vi "Update_Ch_Discription_client.vi"(1 "Channels to update In":T1[](array[typedef]) {"Duty" format="%016b"; "D" format="%#_5g"; "C" format="%#_5g"; "B" format="%#_5g"; "A" format="%#_5g"}) -> ()   [LabVIEW 2016]
doc: "This is an example of using features of the VI Server as a client. It shows how you might browse from one or more applications that may be exporting data from one or more data stations. \n\nThe example shows how to query a server for its list of exported VIs, how to get references to the VIs, and how call them with the Call By Reference function."
uses:
  Anemometry/Anemometry Sub Vis/Globals/Preference_global.vi
  Anemometry/Anemometry Sub Vis/Controls/Global_mode.ctl
  Sub VIs/ADAM Controls/Module_type_ADAM.ctl
  Sub VIs/ADAM Controls/Function_ADAM.ctl
  Sub VIs/ADAM Controls/Calib_type_ADAM.ctl
  Sub VIs/ADAM Controls/Address.ctl
  Sub VIs/ADAM Controls/Ch_description_ADAM.ctl
  Sub VIs/ADAM Controls/Channel_State.ctl
panel:
  in  "Server type":refnum<vi>
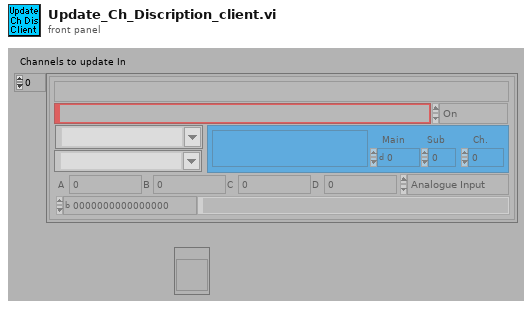
[diagram p1: front panel]
types:
  T1 = typedef "Ch_description_ADAM.ctl" = cluster{"Ch Name":string, "Type":T2, "Function":T3, "Ch State":T4, "Calibration type":T5, "A":dbl, "B":dbl, "C":dbl, "D":dbl, "Comments":string, "Address":T6, "String":string, "Duty":u16}
  T2 = typedef "Module_type_ADAM.ctl" = string
  T3 = typedef "Function_ADAM.ctl" = enum16{"Analogue Input", "Digital Input", "Event counter", "Event rate", "Analogue Output", "Digital Output", "Relay Output"}
  T4 = typedef "Channel_State.ctl" = enum16{"On", "Off", "Always On", "Always Off"}
  T5 = typedef "Calib_type_ADAM.ctl" = string
  T6 = typedef "Address.ctl" = cluster{"Main":i32, "Ch.":i32, "Sub":i32, "Port Name":string}
  T7 = typedef "Server_Comms.ctl" = enum16{"Server Link Healthy", "Do Not Link To Server"}
  T8 = enum16{"Append to Global", "Read Global then Clear"}
  T9 = typedef "Global_mode.ctl" = enum16{"Read Global", "Load Global From File", "Write Global to File"}
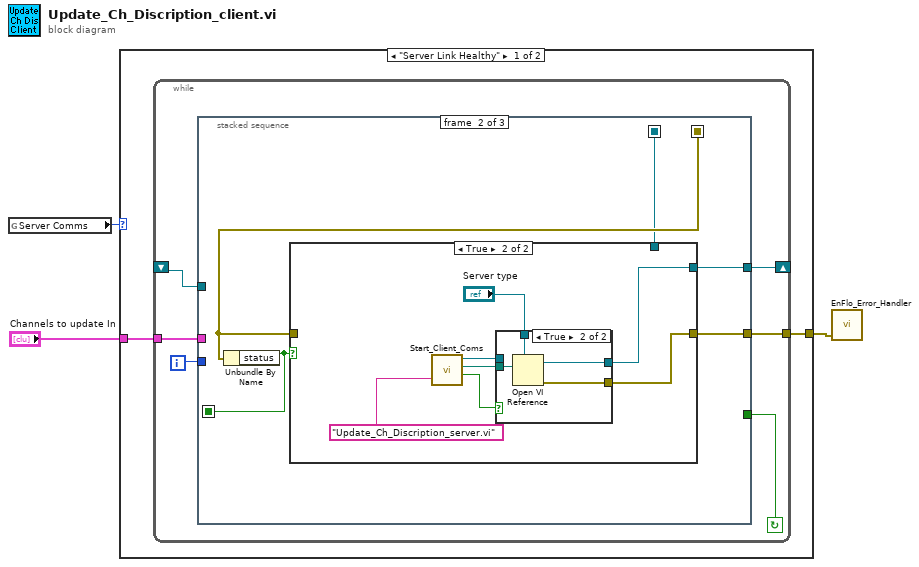
[diagram p0: block diagram]
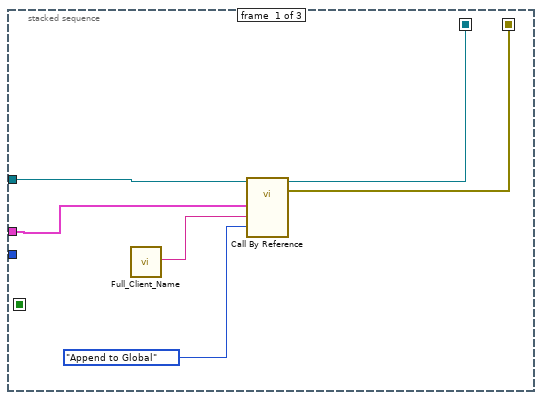
[diagram p2: hidden frame]
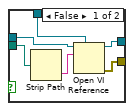
[diagram p4: hidden frame]
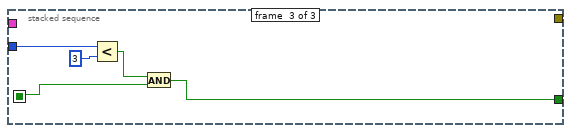
[diagram p5: hidden frame]
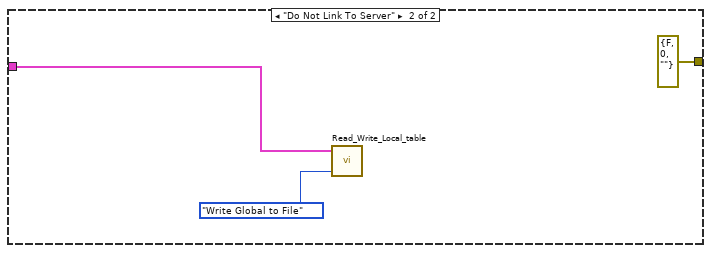
[diagram p6: hidden frame]
diagram:
  n1 = global read "Preference_global.vi" "Server Comms"() -> (w3:T7)
  n2 = case shown="\"Server Link Healthy\"" w3 {
    tunnel: [w5 errorcluster {"status"=FALSE, "code"=0, "source"=""} ("Error IO")] -> w2
    tunnel: "Channels to update In" -> [w4 w47]
    frame "Server Link Healthy" {
      n3 = while {
        tunnel: w4 -> [w7]
        tunnel: [w8] -> w5
        shift-left: _ -> [w11]
        shift-right: [w6] -> _
        i -> [w10]
        stop <- w9 continue-if-true
        n4 = stacked-sequence {
          seq-local: [w12 _ _] -> [_ w18 _]
          seq-local: [w17 _ _] -> [_ w19 _]
          seq-local: [_ w21 _] -> [_ _ w43]
          tunnel: w11 -> [w13 _ _]
          tunnel: [_ w22 _] -> w6
          tunnel: w10 -> [_ _ w44]
          tunnel: [_ _ w42] -> w9
          tunnel: [_ w20 _] -> w8
          tunnel: w7 -> [w14 _ _]
          frame #0 {
            n5 = call "Full_Client_Name.vi"() -> ("Client Name"=w16:string)
            n6 = call-by-ref "?"(reference=w13, "Mode"=T8."Append to Global", "Client HD name"=w16, "Channels to update In"=w14) -> (reference out=w12:refnum<vi>, error out=w17:errorcluster)  [unwired: 1 in, 1 out]
          }
          frame #1 {
            n7 = Unbundle By Name(w19) -> ("status"=w21:bool)
            n8 = case shown="True" w21 {
              tunnel: [w23 w27] -> w22
              tunnel: w18 -> [w23 _]
              tunnel: [w24 w25] -> w20
              tunnel: w19 -> [w24 _]
              frame False {
              }
              frame True {
                n9 = call "Start_Client_Coms.vi"("VI name to run on server"="Update_Ch_Discription_server.vi") -> ("LabVIEW application reference"=w29:refnum<vi>, "Checked VI name"=w30:path, "Local Call"=w28:bool)  [unwired: 1 in, 1 out]
                n10 = case shown="True" w28 {
                  tunnel: [w36 w41] -> w27
                  tunnel: "Server type" -> [w34 w40]
                  tunnel: w30 -> [w33 w39]
                  tunnel: w29 -> [w32 _]
                  tunnel: [w35 w38] -> w25
                  frame False {
                    n11 = Strip Path(path=w33) -> (name=w37:string)  [unwired: 1 out]
                    n12 = Open VI Reference(type specifier VI Refnum (for type only)=w34, application reference (local)=w32, vi path=w37) -> (vi reference=w36:refnum<vi>, error out=w35:errorcluster)  [unwired: 1 in, 2 out]
                  }
                  frame True {
                    n13 = Open VI Reference(type specifier VI Refnum (for type only)=w40, vi path=w39) -> (vi reference=w41:refnum<vi>, error out=w38:errorcluster)  [unwired: 1 in, 3 out]
                  }
                }
              }
            }
          }
          frame #2 {
            n14 = Less?(x=w44, y=3) -> (x < y?=w46:bool)
            n15 = And(x=w46, y=w43) -> (x .and. y?=w42:bool)
          }
        }
      }
    }
    frame "Do Not Link To Server" {
      n16 = call "Read_Write_Local_table.vi"("Mode"=Global_mode."Write Global to File", "Channels Descriptions In"=w47) -> ()  [unwired: 1 in, 3 out]
    }
  }
  n17 = call "EnFlo_Error_Handler.vi"("error in (no error)"=w2) -> ()  [unwired: 2 in, 3 out]
